vi "Change State.vi"(8 "error in (no error)":errorcluster, 10 "Input":string, 11 "StateMachine in":refnum<class "StateMachine.lvclass">) -> (0 "error out":errorcluster, 2 "Output State":string, 3 "StateMachine out":refnum<class "StateMachine.lvclass">)   [LabVIEW 2018, in "State Machine.lvlib" / "StateMachine.lvclass"]
doc: "This VI manages the state transitions from the data in the state machine class."
uses:
  StateMachine.lvclass
  StateMachine.lvclass/StateMachine.ctl
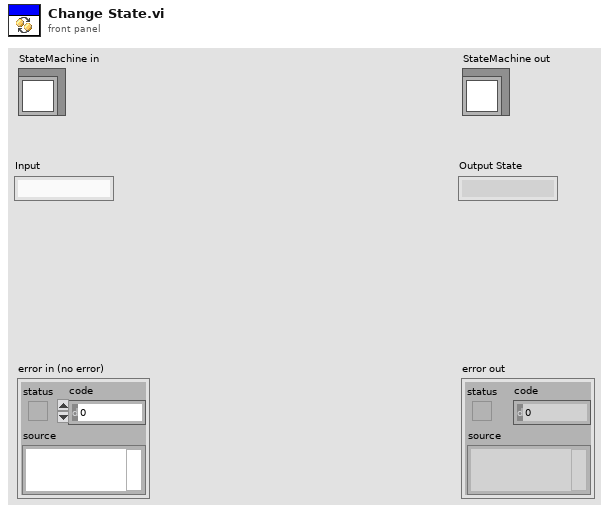
[diagram p1: front panel]
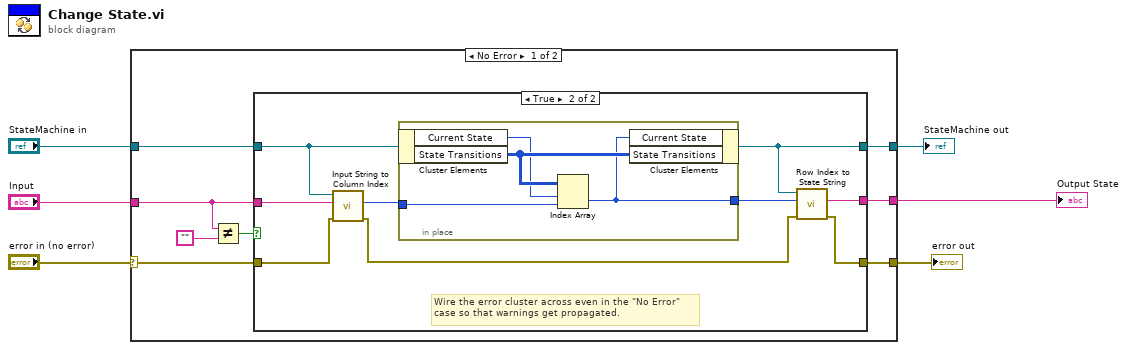
[diagram p0: block diagram]
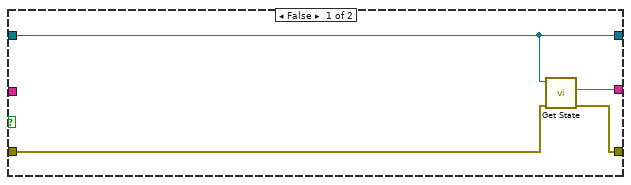
[diagram p2: hidden frame]
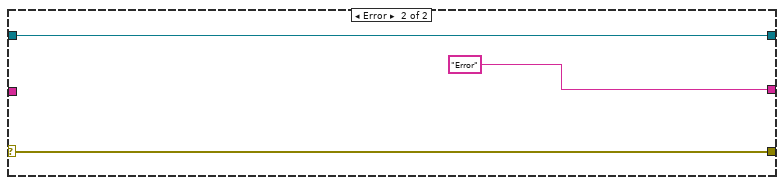
[diagram p3: hidden frame]
diagram:
  n1 = case shown="No Error" "error in (no error)" {
    selector: "error in (no error)" -> [w11 w34]
    tunnel: [w10 w34] -> w5
    tunnel: [w13 w33] -> w3
    tunnel: "StateMachine in" -> [w14 w33]
    tunnel: "Input" -> [w8 _]
    tunnel: [w12 "Error" ("String")] -> w1
    frame No Error {
      n2 = Not Equal?(x=w8, y="") -> (x != y?=w9:bool)
      n3 = case shown="True" w9 {
        tunnel: w14 -> [w17 w27]
        tunnel: w8 -> [_ w26]
        tunnel: [w17 w23] -> w13
        tunnel: [w18 w22] -> w12
        tunnel: w11 -> [w15 w21]
        tunnel: [w16 w19] -> w10
        frame False {
          n4 = call-dynamic "Get State.vi"("error in (no error)"=w15, "StateMachine in"=w17) -> ("error out"=w16:errorcluster, "State"=w18:string)  [unwired: 7 in, 1 out]
        }
        frame True {
          # "Wire the error cluster across even in the \"No Error\"\ncase so that warnings get propagated."
          n5 = call-dynamic "Input String to Column Index.vi"("error in (no error)"=w21, "Input String"=w26, "StateMachine in"=w27) -> ("error out"=w20:errorcluster, "Column Index"=w25:i32)  [unwired: 6 in, 1 out]
          n6 = in-place {
            in-place-border: w25 -> [w29]
            in-place-border: [w28] -> w24
            n7 = in-place-cluster #1(w27) -> ("Current State"=w30:i32, "State Transitions"=w31:i32[][])
            n8 = Index Array(array=w31, index (row)=w30, index (col)=w29) -> (element=w28:i32)
            n9 = in-place-cluster #1("Current State"=w28, "State Transitions"=w31) -> (w23:refnum<class "StateMachine.lvclass">)
          }
          n10 = call-dynamic "Row Index to State String.vi"("error in (no error)"=w20, "Row Index"=w24, "StateMachine in"=w23) -> ("error out"=w19:errorcluster, "State String"=w22:string)  [unwired: 6 in, 1 out]
        }
      }
    }
    frame Error {
    }
  }
  "error out" <- w5
  "StateMachine out" <- w3
  "Output State" <- w1
